vi "Create Process Event Registration.vi"(8 "error in (no error)":errorcluster, 11 "SMO in":refnum<class "SMO.lvclass">) -> (0 "error out":errorcluster, 3 "SMO out":refnum<class "SMO.lvclass">)   [LabVIEW 2013, in "SMO.lvclass"]
uses:
  SMO.lvclass
  Typedefs/SMOState --Enum.ctl
  Support/Attribute.Owner/Packet -- Cluster.ctl
  Typedefs/ProcessRegistrationRefnum.ctl
  Typedefs/AbortProcessEventData--Cluster.ctl
  Typedefs/StopProcessEventData--Cluster.ctl
  Typedefs/SMO Dependency Event--Cluster.ctl
  Typedefs/SMO Dependency Event--Enum.ctl
  SMO.lvclass/SMO.ctl
  Support/Attribute.Owner/Attribute.Owner.lvclass
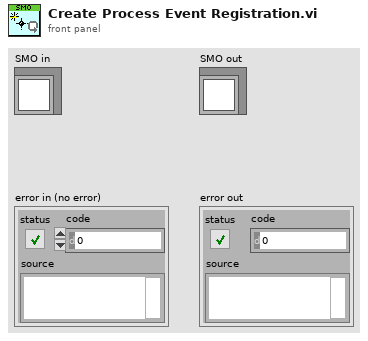
[diagram p1: front panel]
types:
  T1 = typedef "SMO.lvclass/ProcessRegistrationRefnum.ctl" = refnum<event-registration>
  T2 = typedef "SMO.lvclass/Protected Events.ctl" = cluster{"StopProcesses":refnum<user-event>, "AbortProcesses":refnum<user-event>, "Config Changed":refnum<user-event>, "Dependency":refnum<user-event>}
  T3 = typedef "SMO.lvclass/Public Events.ctl" = cluster{"Error":refnum<user-event>, "State":refnum<user-event>, "Reserve State":refnum<user-event>}
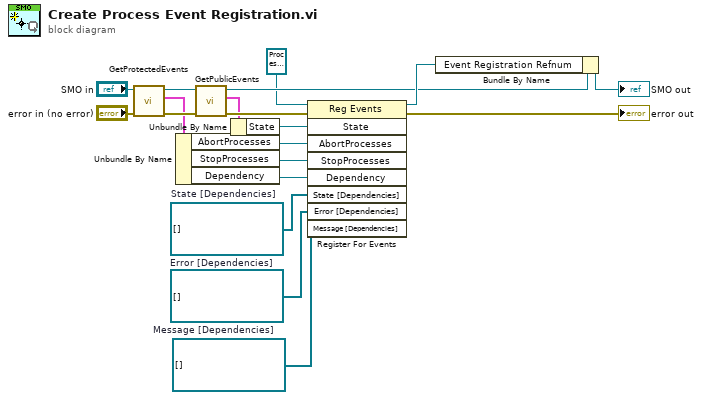
[diagram p0: block diagram]
diagram:
  w19 = refnum<user-event>[] []  # Message [Dependencies]
  w18 = refnum<user-event>[] []  # Error [Dependencies]
  w15 = refnum<user-event>[] [] items=["unknown", "Created", "Started", "Stopped"]  # State [Dependencies]
  n1 = call "GetProtectedEvents.vi"("error in (no error)"="error in (no error)", "SMO"="SMO in") -> ("error out"=w10:errorcluster, "SMO Protected Events"=w7:T2, "SMO out"=w9:refnum<class "SMO.lvclass">)  [unwired: 7 in]
  n2 = Unbundle By Name(w7) -> ("AbortProcesses"=w6:refnum<user-event>, "StopProcesses"=w12:refnum<user-event>, "Dependency"=w14:refnum<user-event>)
  n3 = call "GetPublicEvents.vi"("error in (no error)"=w10, "SMO"=w9) -> ("error out"=w11:errorcluster, "Public Events"=w8:T3, "SMO out"=w3:refnum<class "SMO.lvclass">)  [unwired: 7 in]
  n4 = Unbundle By Name(w8) -> ("State"=w5:refnum<user-event>)
  n5 = register-events(reference=T1 refnum ("Event Registration Refnum"), error in=w11, w5, w6, w12, w14, w15, w18, w19) -> (reference out=w4:T1, error out=→"error out":errorcluster)
  n6 = Bundle By Name(cluster=w3, "Event Registration Refnum"=w4) -> (→"SMO out":refnum<class "SMO.lvclass">)
